vi "0x56_Cmd_freeing_data_from_a_prepared_table_parameter_(SubVI).vi"(10 "Parameters":cluster{"Номер табличного параметра":i32}, 11 "String in":string) -> (3 "String out":string)   [LabVIEW 2017, in "LV_Unicorn.lvlib"]
uses:
  LV_Unicorn.lvlib
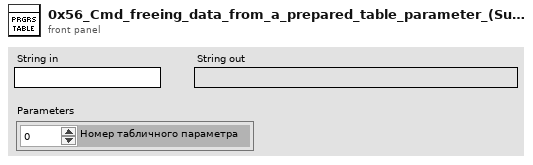
[diagram p1: front panel]
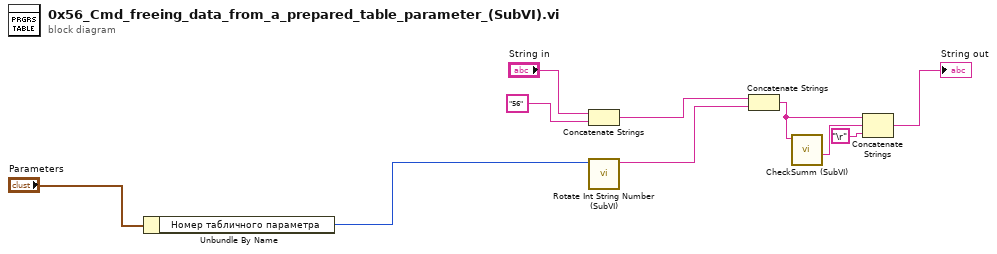
[diagram p0: block diagram]
diagram:
  n1 = Unbundle By Name("Parameters") -> ("Номер табличного параметра"=w2:i32)
  n2 = Concatenate Strings("String in", "56" ("string")) -> (w8:string)
  n3 = call "Rotate Int String Number (SubVI).vi"("Int Number In"=w2) -> ("Orig String"=w3:string)  [unwired: 8 in, 2 out]
  n4 = Concatenate Strings(w8, w3) -> (w5:string)
  n5 = call "CheckSumm (SubVI).vi"("Input String"=w5) -> ("CheckSumm"=w4:string)  [unwired: 7 in, 3 out]
  n6 = Concatenate Strings(w5, w4, "\r") -> (→"String out":string)
